vi "Update LEDs.vi"   [LabVIEW 2012]
uses:
  Globals/Useful Values.vi
types:
  T1 = typedef "WPI_RelayDevRef.ctl" = cluster{"DevStatus":errorcluster, "Relay Channel":T2, "Digital Module":T3, "Relay Direction":T4}
  T2 = typedef "FPGA_DIORelayChannel.ctl" = enum8{"Relay 1", "Relay 2", "Relay 3", "Relay 4", "Relay 5", "Relay 6", "Relay 7", "Relay 8", "Invalid"}
  T3 = typedef "FPGA_TypedefDigitalModule.ctl" = enum16{"Digital Module 1", "Digital Module 2"}
  T4 = typedef "WPI_RelayDirection.ctl" = enum16{"Both directions", "Forward only", "Reverse only"}
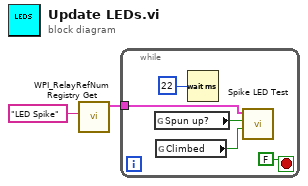
[diagram p0: block diagram]
diagram:
  n1 = call <vilib>:"WPI_RelayRefNum Registry Get.vi"("refnum name"="LED Spike" ("Spike")) -> ("RelayDevRef"=w1:T1)  [unwired: 9 in, 1 out]
  n2 = while {
    tunnel: w1 -> [w5]
    stop <- FALSE stop-if-true
    n3 = global read "Useful Values.vi" "Spun up?"() -> (w6:bool)
    n4 = global read "Useful Values.vi" "Climbed"() -> (w3:bool)
    n5 = Wait (ms)(milliseconds to wait=u32 22) -> ()  [unwired: 1 out]
    n6 = call "Spike LED Test.vi"("Climb"=w3, "Spun up"=w6, "Spike"=w5) -> ()  [unwired: 9 in]
  }
